vi "DAQ 1SDI v02.vi"() -> ()   [LabVIEW 2013]
uses:
  <instrlib>/niScope/Controls/niScope vertical coupling.ctl
  Strict Type Defs/type_meas_enum.ctl
  Strict Type Defs/Monitor switches.ctl
  Global VIs/shotnoise.vi
panel:
  in  "Monitors":T1(tab)=enum."Monitors On 2"
  out "Variance 1 normalised to SNL":dbl(graph)=0.20510373274335536
  out "Conditional variance":dbl(graph)=1.0471612982510168
  out "Variance 2 normalised to SNL":dbl(graph)=0.2270313335820158
  out "covariance":dbl(graph)=0.035536693140327605
  out "covariance A|B":dbl(graph)=-0.012388635851318691
  out "Conditional variance A|B":dbl(graph)=1.0856496659797459
  out "Key rate A|B":dbl(graph)=-0.5612536682540186
  out "Loop count":i32=1920
  in  "stop":bool
  in  "Settings":enum32{"Settings and Record", "Under the hood"}(tab)
  out "Video bandwidth (Hz)":dbl=666.6666666666666
  in  "Minimum sample rate (S/s)":dbl=20000000.0 format="%#_6p"
  in  "Reference position":dbl(slide)=50.0 scale=0.0..100.0
  in  "max time (s)":dbl=10.0 caption="Time to run (s)"
  in  "Channel parameters":T3(array[cluster])=[{"Channel name"="0", "Input impedance (Ohms)"=2, "Maximum input frequency (Hz)"=10000000.0, "vertical coupling"=1, "Probe attenuation"=1.0, "Vertical range (V)"=0.5, "Vertical offset"=0.0, "channel enabled"=TRUE}, {"Channel name"="1", "Input impedance (Ohms)"=2, "Maximum input frequency (Hz)"=10000000.0, "vertical coupling"=1, "Probe attenuation"=1.0, "Vertical range (V)"=0.5, "Vertical offset"=0.0, "channel enabled"=TRUE}] {"Input impedance (Ohms)" items=["1 mega ohm"=0, "50 ohms"=2]; "Maximum input frequency (Hz)" format="%#_6p"; "vertical coupling" items=["AC", "DC", "Ground"]}
  in  "IIR filter specifications":T4={"Topology"=enum."Butterworth", "Type"=enum."Bandpass", "Order"=6, "Lower Fc"=2900000.0, "Upper Fc"=3100000.0, "PB Ripple"=1.0, "SB Attenuation"=60.0} {"PB Ripple" format="%0.2f"; "SB Attenuation" format="%0.2f"; "Lower Fc" format="%0.2p"; "Upper Fc" format="%0.2p"}
  in  "File location":path=path "C:/ni-rt/LabVIEW Data/June17"
  in  "Record Data":bool
  in  "Type of measurement":T5
  in  "File root name":string="Optimal_2_21"
  in  "Number of samples 2":i32=30000 format="%.0p"
  in  "reset sn":bool
  in  "Shot noise start":bool
  out "error out":errorcluster caption="error out final"
  in  "Additional text":string="OPA 1 optical power set to 15mV on HD A.\nOPA 2 optical power set to 15mV on HD B.\nLocal oscillator is set to 5V on HD.\nParametric gain set to 15 for OPA 1.\nParametric gain set to 15 for OPA 2.\nVertical range set to 0.5V for both channels.\nSample rate set to 20MS/s.\nMax input freq set to 10MHz.\nVisibility between OPA 1 & OPA 2 = 99.7\nVisibility between OPA 1 & L.O. 1 = 99.0\nVisibility between OPA 1 & L.O. 2 = 99.0\nBoth squeezers expected to produce -7dB/11dB.\n\n\n"
  out "Actual samples acquired ch 0":i32=30000
  out "Actual samples acquired ch 1":i32=30000
  out "SN loop count":i64=58
  out "SN":dbl[](array[numeric])=[0.005851578758312275, 0.005592280462681344]
  out "Parameters values file":string="PARAMETERS VALUES\r\rTuesday, June 17, 2014\r7:02 PM\r\rMaster ch 0 <-> HD1 AC a-b\nMaster ch 1 <-> HD2 AC a-b\n\rSample rate : \rMaster : 20.000000E+6 Samples per second\rNumber of samples :\rMaster ch 0 : 30.000000E+3\rMaster ch 1 : 30.000000E+3\rFiles names : \rOptimal_2_21_shot_ParametersValues_30000.txt\rOptimal_2_21_shot_mch01_60000.txt\r\rOPA 1 optical power set to 15mV on HD A.\nOPA 2 optical power set to 15mV on HD B.\nLocal oscillator is set to 5V on HD.\nParametric gain set to 15 for OPA 1.\nParametric gain set to 15 for OPA 2.\nVertical range set to 0.5V for both channels.\nSample rate set to 20MS/s.\nMax input freq set to 10MHz.\nVisibility between OPA 1 & OPA 2 = 99.7\nVisibility between OPA 1 & L.O. 1 = 99.0\nVisibility between OPA 1 & L.O. 2 = 99.0\nBoth squeezers expected to produce -7dB/11dB.\n\n\n"
  in  "DAQ Card":refnum<k15>="PXI1Slot7"
  in  "Monitor Switches":T6
  # "Variance won't be displayed until shot noise is taken"
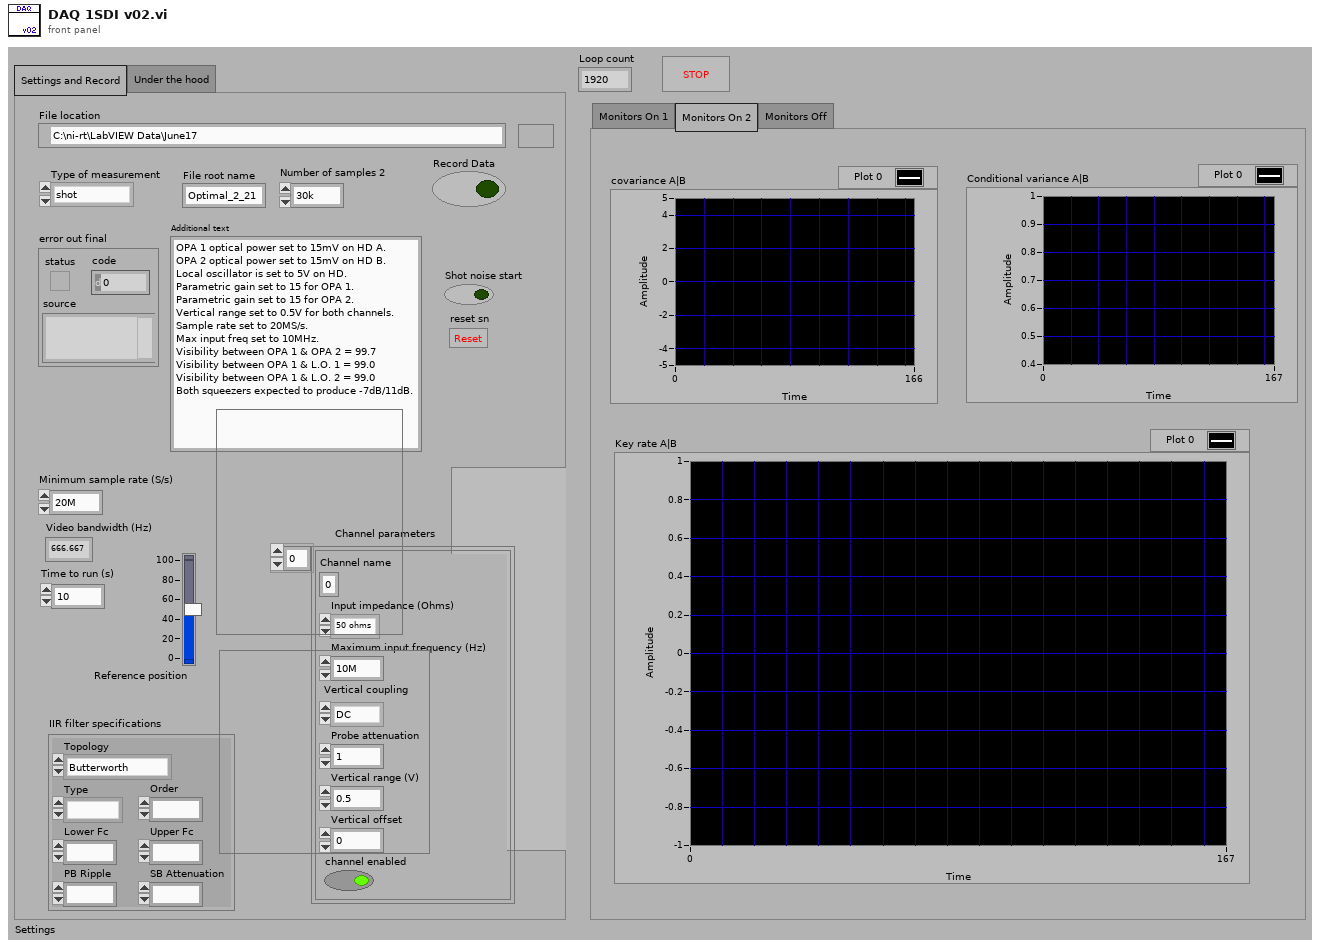
[diagram p1: front panel]
types:
  T1 = enum32{"Monitors On 1", "Monitors On 2", "Monitors Off"}
  T2 = typedef "niScope vertical coupling.ctl" = i32
  T3 = cluster{"Channel name":string, "Input impedance (Ohms)":u32, "Maximum input frequency (Hz)":dbl, "vertical coupling":T2, "Probe attenuation":dbl, "Vertical range (V)":dbl, "Vertical offset":dbl, "channel enabled":bool}[]
  T4 = cluster{"Topology":enum16{"Off", "Butterworth", "Chebyshev", "Inverse Chebyshev", "Elliptic", "Bessel"}, "Type":enum16{"Lowpass", "Highpass", "Bandpass", "Bandstop"}, "Order":i32, "Lower Fc":dbl, "Upper Fc":dbl, "PB Ripple":dbl, "SB Attenuation":dbl}
  T5 = typedef "type_meas_enum.ctl" = enum16{"shot", "x", "p", "electronic"}
  T6 = typedef "Monitor switches.ctl" = cluster{"Signal 1 On":bool, "Signal 2 On":bool, "Variance 1 On":bool, "Variance 2 On":bool, "Cov On":bool, "Cond. On":bool, "Monitors On":bool}
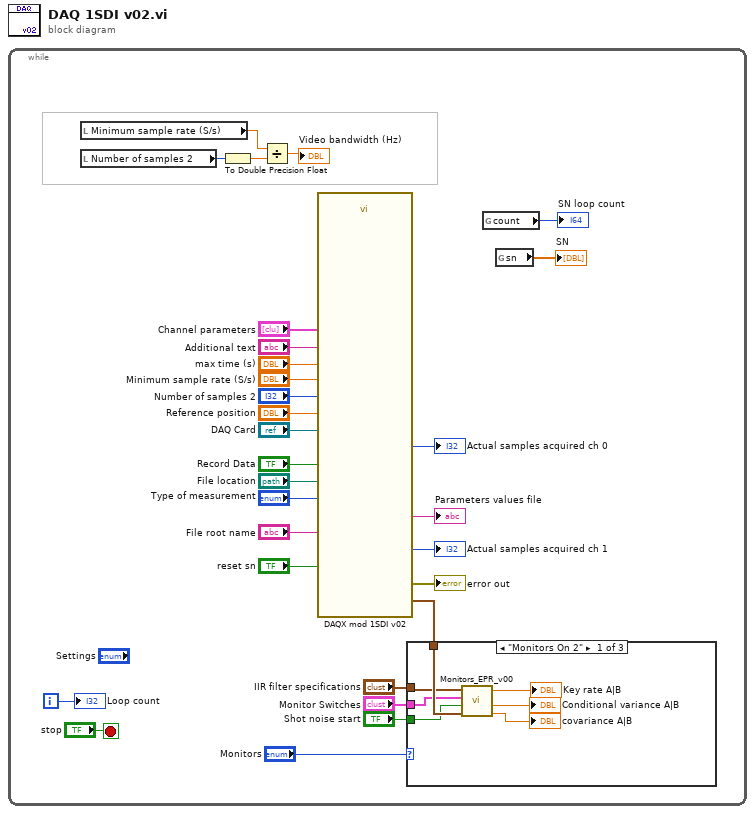
[diagram p0: block diagram]
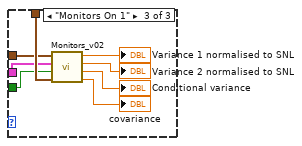
[diagram p3: hidden frame]
diagram:
  n1 = while {
    i -> [w11]
    stop <- "stop" stop-if-true
    n2 = local read "Minimum sample rate (S/s)"() -> (w27:dbl)
    n3 = local read "Number of samples 2"() -> (w29:i32)
    n4 = To Double Precision Float(number=w29) -> (double precision float=w26:dbl)
    n5 = Divide(x=w27, y=w26) -> (x/y=→"Video bandwidth (Hz)":dbl)
    n6 = call "DAQX mod 1SDI v02.vi"("resource name"="DAQ Card", "Record Data"="Record Data", "numSamples"="Number of samples 2", "max time (s)"="max time (s)", "min sample rate"="Minimum sample rate (S/s)", "File location"="File location", "reference position"="Reference position", "Additional text"="Additional text", "Type of measurement"="Type of measurement", "Name root"="File root name", "channel parameters"="Channel parameters", "reset sn"="reset sn") -> ("wfm out"=w7:waveform(dbl)[], "Parameters values file"=→"Parameters values file":string, "actualSamples 0"=→"Actual samples acquired ch 0":i32, "actualSamples 1"=→"Actual samples acquired ch 1":i32, "error out"=→"error out":errorcluster)  [unwired: 11 in]
    n7 = case shown="\"Monitors On 2\"" "Monitors" {
      tunnel: w7 -> [w34 _ w44]
      tunnel: "IIR filter specifications" -> [w33 _ w39]
      tunnel: "Monitor Switches" -> [w32 _ w38]
      tunnel: "Shot noise start" -> [w31 _ w37]
      frame "Monitors On 2" {
        n8 = call "Monitors_EPR_v00.vi"("wfm"=w34, "Shot noise start"=w31, "Monitor Switches"=w32, "IIR filter specifications"=w33) -> ("covariance"=→"covariance A|B":dbl, "conditional variance A|B"=→"Conditional variance A|B":dbl, "Key Rate A|B"=→"Key rate A|B":dbl)  [unwired: 5 in]
      }
      frame "Monitors Off" {
      }
      frame "Monitors On 1" {
        n9 = call "Monitors_v02.vi"("wfm"=w44, "Shot noise start"=w37, "Monitor Switches"=w38, "IIR filter specifications"=w39) -> ("covariance"=→"covariance":dbl, "conditional variance"=→"Conditional variance":dbl, "Variance 2 normalised to SNL"=→"Variance 2 normalised to SNL":dbl, "Variance 1 normalised to SNL"=→"Variance 1 normalised to SNL":dbl)  [unwired: 4 in]
      }
    }
    n10 = global read "shotnoise.vi" "count"() -> (→"SN loop count":i64)
    n11 = global read "shotnoise.vi" "sn"() -> (→"SN":dbl[])
    "Loop count" <- w11
  }
